vi "AB_RW_Non_Persistent_Tags.vi"(7 "action":T3, 8 "error in (no error)":errorcluster, 10 "data in":T1, 11 "buildObject":T2) -> (0 "error out":errorcluster, 2 "data out":T1, 3 "buildObject out":T2)   [LabVIEW 2020]
doc: "Reads and writes the data to the object property bag."
uses:
  <resource>/Framework/Providers/API/ItemRef.ctl
  <vilib>/AppBuilder/RW_Project/AB_RW_Project_PropBag_Action.ctl
  <vilib>/AppBuilder/RW_Project/AB_RW_Non_Persistent_Data.ctl
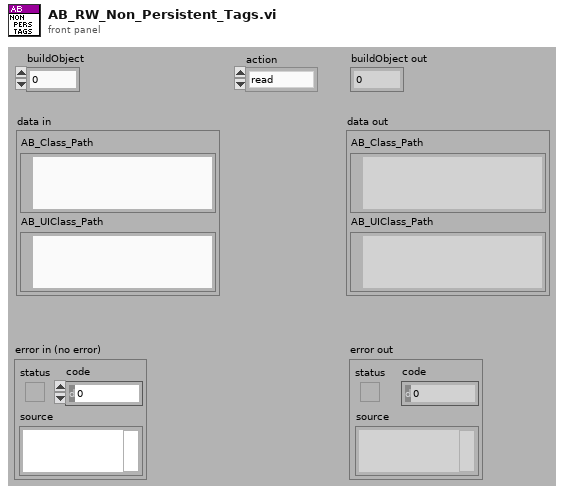
[diagram p1: front panel]
types:
  T1 = typedef "AB_RW_Non_Persistent_Data.ctl" = cluster{"AB_Class_Path":path, "AB_UIClass_Path":path}
  T2 = typedef "ItemRef.ctl" = u64
  T3 = typedef "AB_RW_Project_PropBag_Action.ctl" = enum16{"read", "write", "clear", "readPrevious", "writePrevious", "clearPrevious"}
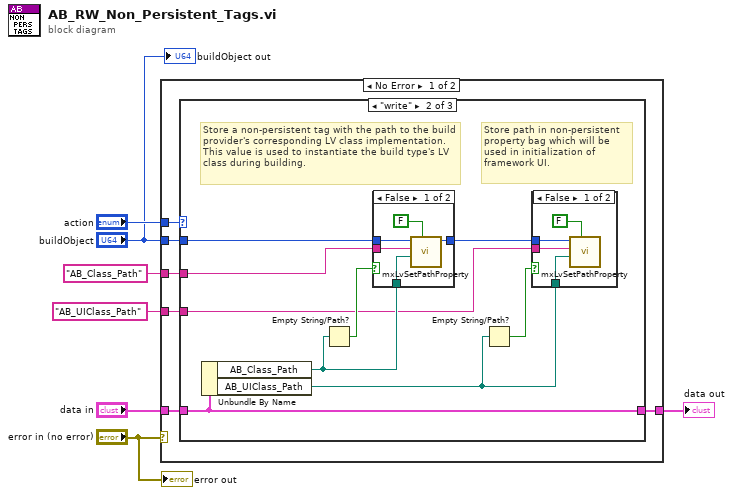
[diagram p0: block diagram]
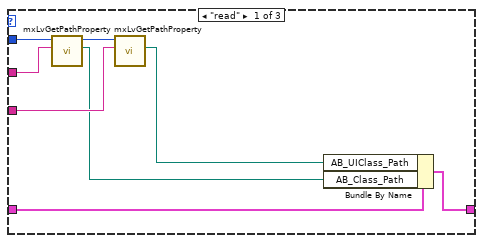
[diagram p2: hidden frame]
diagram:
  n1 = case shown="No Error" "error in (no error)" {
    tunnel: "action" -> [w13 _]
    tunnel: "buildObject" -> [w12 _]
    tunnel: "data in" -> [w11 w42]
    tunnel: "AB_Class_Path" ("Tag") -> [w10 _]
    tunnel: [w9 w42] -> w1
    tunnel: "AB_UIClass_Path" ("Tag") -> [w8 _]
    frame No Error {
      n2 = case shown="\"write\"" w13 {
        tunnel: w12 -> [w21 w30 _]
        tunnel: w11 -> [w17 w28 w41]
        tunnel: w10 -> [w20 w29 _]
        tunnel: [w14 w28 w41] -> w9
        tunnel: w8 -> [w18 w24 _]
        frame "read" {
          n3 = call <resource>:"mxLvGetPathProperty.vi"("Tag"=w20, "Item"=w21) -> ("Path"=w16:path, "Item"=w19:T2)  [unwired: 2 in, 6 out]
          n4 = call <resource>:"mxLvGetPathProperty.vi"("Tag"=w18, "Item"=w19) -> ("Path"=w15:path)  [unwired: 2 in, 7 out]
          n5 = Bundle By Name(cluster=w17, "AB_UIClass_Path"=w15, "AB_Class_Path"=w16) -> (w14:T1)
        }
        frame "write" {
          # "Store path in non-persistent property bag which will be used in initialization of framework UI."
          # "Store a non-persistent tag with the path to the build provider's corresponding LV class implementation. This value is used to instantiate the build type's LV class during building."
          n6 = Unbundle By Name(w28) -> ("AB_Class_Path"=w27:path, "AB_UIClass_Path"=w23:path)
          n7 = Empty String/Path?(string/path=w27) -> (empty?=w26:bool)
          n8 = case shown="False" w26 {
            tunnel: w30 -> [w39 w40]
            tunnel: w29 -> [w38 _]
            tunnel: [w36 w40] -> w25
            tunnel: w27 -> [w35 _]
            frame False {
              n9 = call <resource>:"mxLvSetPathProperty.vi"("Persist Property? (T)"=FALSE, "Path"=w35, "Tag"=w38, "Item"=w39) -> ("Item"=w36:T2)  [unwired: 1 in, 6 out]
            }
            frame True {
            }
          }
          n10 = Empty String/Path?(string/path=w23) -> (empty?=w22:bool)
          n11 = case shown="False" w22 {
            tunnel: w25 -> [w34 _]
            tunnel: w24 -> [w33 _]
            tunnel: w23 -> [w31 _]
            frame False {
              n12 = call <resource>:"mxLvSetPathProperty.vi"("Persist Property? (T)"=FALSE, "Path"=w31, "Tag"=w33, "Item"=w34) -> ()  [unwired: 1 in, 7 out]
            }
            frame True {
            }
          }
        }
        frame "clear", Default {
        }
      }
    }
    frame Error {
    }
  }
  "data out" <- w1
  "error out" <- "error in (no error)"
  "buildObject out" <- "buildObject"
